vi "文件IO.vi"() -> ()   [LabVIEW 2014]
panel:
  in  "停止":bool
  out "数值 2":dbl
  out "数值":dbl
  in  "旋钮 2":dbl(knob) scale=0.0..10.0
  in  "旋钮":dbl(knob) scale=0.0..10.0
  out "字符串显示":string
  in  "字符串写入":string
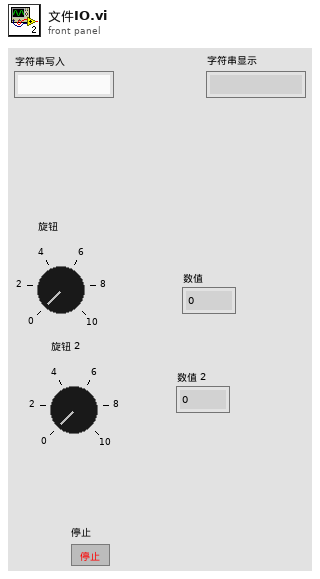
[diagram p1: front panel]
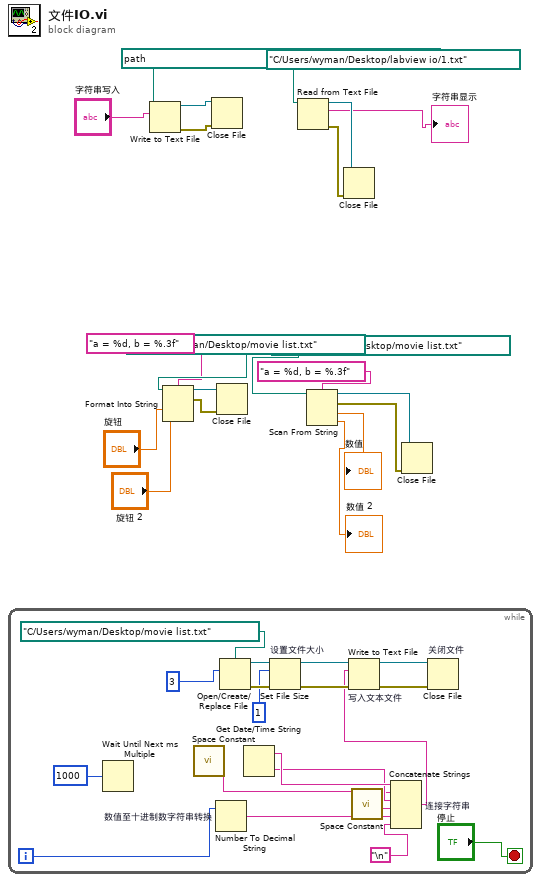
[diagram p0: block diagram]
diagram:
  n1 = while {
    i -> [w32]
    stop <- "停止" stop-if-true
    n2 = Wait Until Next ms Multiple(millisecond multiple=1000) -> ()  [unwired: 1 out]
    n3 = call <vilib>:"Space Constant.vi"() -> ("String"=w24:string)
    n4 = Number To Decimal String "数值至十进制数字符串转换"(number=w32) -> (decimal integer string=w28:string)  [unwired: 1 in]
    n5 = Open/Create/Replace File(file path (use dialog)=path "C:/Users/wyman/Desktop/movie list.txt" ("路径"), operation (0:open)=3) -> (refnum out=w36:refnum<file>, error out=w38:errorcluster)  [unwired: 4 in, 1 out]
    n6 = Get Date/Time String() -> (date string=w26:string, time string=w25:string)  [unwired: 3 in]
    n7 = Set File Size "设置文件大小"(4:w38, 6:1, 7:w36) -> (0:w39:errorcluster, 3:w35:refnum<file>)
    n8 = call <vilib>:"Space Constant.vi"() -> ("String"=w27:string)
    n9 = Concatenate Strings "连接字符串"(w26, w24, w25, w27, w28, "\n") -> (w22:string)
    n10 = Write to Text File "写入文本文件"(file (use dialog)=w35, text=w22, error in=w39) -> (refnum out=w34:refnum<file>, error out=w37:errorcluster)  [unwired: 1 in, 1 out]
    n11 = Close File "关闭文件"(refnum=w34, error in=w37) -> ()  [unwired: 2 out]
  }
  n12 = Write to Text File(file (use dialog)=path "C:/Users/wyman/Desktop/labview io/新建文本文档.txt" ("路径"), text="字符串写入") -> (refnum out=w19:refnum<file>, error out=w18:errorcluster)  [unwired: 2 in, 1 out]
  n13 = Format Into String(format string="a = %d, b = %.3f", initial string=path "C:/Users/wyman/Desktop/movie list.txt" ("路径"), "旋钮", "旋钮 2") -> (resulting string=w12:refnum<file>, error out=w11:errorcluster)  [unwired: 1 in]
  n14 = Close File(refnum=w19, error in=w18) -> ()  [unwired: 2 out]
  n15 = Close File(refnum=w12, error in=w11) -> ()  [unwired: 2 out]
  n16 = Read from Text File(file (use dialog)=path "C:/Users/wyman/Desktop/labview io/1.txt" ("路径")) -> (refnum out=w16:refnum<file>, text=→"字符串显示":string, error out=w17:errorcluster)  [unwired: 3 in, 1 out]
  n17 = Scan From String("a = %d, b = %.3f", path "C:/Users/wyman/Desktop/movie list.txt" ("路径")) -> (w5:refnum<file>, w6:errorcluster, output 1=→"数值":dbl, output 2=→"数值 2":dbl)  [unwired: 3 in]
  n18 = Close File(refnum=w16, error in=w17) -> ()  [unwired: 2 out]
  n19 = Close File(refnum=w5, error in=w6) -> ()  [unwired: 2 out]
